vi "CountTo10.vi"() -> ()   [LabVIEW 2012]
panel:
  out "Numeric":i32
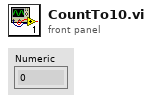
[diagram p1: front panel]
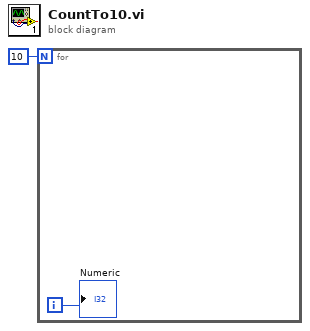
[diagram p0: block diagram]
diagram:
  n1 = for {
    N: 10 -> [_]
    i -> [w2]
    "Numeric" <- w2
  }
